vi "sv_Harmonic Distortion and Noise.vi"(0 "complex spectrum":T11={"complex spectrum response"={"f0"=0.0, "df"=1.0, "complex spectrum"=[]}, "spectrum info"={"channel name"="", "description"="", "x-axis units"=0, "spectral info"={"spectrum type"=enum."Power [Magnitude^2]", "linear/dB"=enum."linear", "window"=0, "window size"=0, "FFT size"=0}, "engineering units"=0, "custom label"="", "dB reference [EU]"=0.0, "peak units"=enum."rms", "weighting filter"=0, "spectral density?"=FALSE, "unit label"="", "spectrum skewed?"=FALSE, "complimentary spectrum units"=enum."none"}} {"spectrum info"."x-axis units" items=["Time (s)"=0, "Frequency-CB (Hz)"=1, "Frequency-CPB (Hz)"=1248, "Frequency-Arbitrary (Hz)"=2357, "Quefrency (s)"=2, "Revolutions (rev)"=3, "Order"=4, "Speed (RPM)"=11, "Speed (rad/s)"=21, "Index"=65535]; "spectrum info"."weighting filter" items=["Linear", "A-weighting", "B-weighting", "C-weighting", "ITU-R 468-4", "Dolby", "CCITT", "C-message", "Wb", "Wc", "Wd", "We", "Wf", "Wh", "Wj", "Wk", "Wm", "AES17 20 kHz lowpass", "AES17 40 kHz lowpass", "AES17 20 kHz highpass", "AES17 40 kHz highpass"]; "spectrum info"."dB reference [EU]" format="%.2f"; "spectrum info"."engineering units" items=["custom..."=0, "V"=1, "A"=21, "C"=30, "pC"=31, "s"=32, "-"=29, "Pa"=2, "N"=20, "g"=3, "m/s^2"=4, "m/s"=5, "m"=6, "mm/s"=12, "mm"=13, "micron/s"=14, "micron"=15, "in/s^2"=7, "in/s"=8, "in"=9, "mil/s"=10, "mil"=11, "rad/s^2"=16, "rad/s"=17, "rad"=18, "deg/s^2"=26, "deg/s"=27, "deg"=28, "RPM"=22, "cycle/s^2"=23, "Hz"=24, "cycle"=25, "strain"=19]; "spectrum info"."spectral info"."window" items=["None "=0, "Hanning"=1, "Hamming"=2, "Blackman-Harris"=3, "Exact Blackman"=4, "Blackman"=5, "Flat Top"=6, "4 Term B-Harris "=7, "7 Term B-Harris"=8, "Low Sidelobe"=9, "Force - Exponential"=10, "Gaussian"=62]; "complex spectrum response"."complex spectrum" format="%.2f"; "complex spectrum response"."df" format="%.2f"; "complex spectrum response"."f0" format="%.2f"}, 3 "frequency range":T4={"start frequency"=-1.0, "stop frequency"=-1.0} {"stop frequency" format="%.2f"; "start frequency" format="%.2f"}, 4 "advanced span [Hz]":dbl=-1.0 format="%.2f", 5 "error in":errorcluster, 8 "maximum harmonic":i32=5, 9 "approx. fund. freq. (optional)":dbl=-1.0 format="%.2p") -> (10 "actual maximum harmonic":i32=5, 11 "detected fundamental frequency":dbl=nan format="%.3p", 12 "frequency range string":string, 13 "detected amplitude":dbl=nan format="%.3p", 15 "distortion measurements":T2={"SINAD [ratio]"=nan, "THD+N [ratio]"=nan, "THD"=nan} {"THD" format="%.3p"; "THD+N [ratio]" format="%.3p"; "SINAD [ratio]" format="%.3p"}, 16 "energy":T1={"total"=nan, "fundamental"=nan, "noise and harmonics"=nan, "harmonic energy"=nan, "noise"=nan} {"noise" format="%.3p"; "harmonic energy" format="%.3p"; "noise and harmonics" format="%.3p"; "fundamental" format="%.3p"; "total" format="%.3p"}, 17 "harmonic components":T3(array[cluster]) {"detected amplitude" format="%.2f"; "detected frequency [Hz]" format="%.2f"}, 19 "error out":errorcluster)   [LabVIEW 2017, in "SoundVib_Distortion.lvlib"]
uses:
  <vilib>/addons/Sound and Vibration/svt_Distortion/SoundVib_Distortion.lvlib
  <vilib>/addons/_NISVFA/_Shared subVIs/Controls/svc_Spectrum Info.ctl
  <vilib>/addons/_NISVFA/_Shared subVIs/Controls/svc_X-Axis Units.ctl
  <vilib>/addons/_NISVFA/_Shared subVIs/Controls/svc_Spectrum Type.ctl
  <vilib>/addons/_NISVFA/_Shared subVIs/Controls/svc_Engineering Units Text Ring.ctl
  <vilib>/addons/_NISVFA/_Shared subVIs/Controls/svc_Weighting Filter Text Ring.ctl
  <vilib>/addons/_NISVFA/_Shared subVIs/Controls/svc_Complimentary Spectrum Units.ctl
  <vilib>/Analysis/BLAS.llb/nrm2 - Vector 2-Norm.vi
  <vilib>/Analysis/BLAS.llb/dznrm2 - Vector 2-Norm (CDB).vi
  <vilib>/addons/_NISVFA/_Shared subVIs/Common/svc_Convert Start and Stop to Start Index and Length.vi
  <vilib>/addons/_NISVFA/_Shared subVIs/Common/svc_Window Parameters.vi
  <vilib>/addons/_NISVFA/_Spectrum Processing/subVIs/svfa_Spectrum Info Window to windowTd Type Def.vi
  <vilib>/addons/_NISVFA/_Spectrum Processing/SVFA Get Spectrum Subset (Complex) (1 Ch).vi
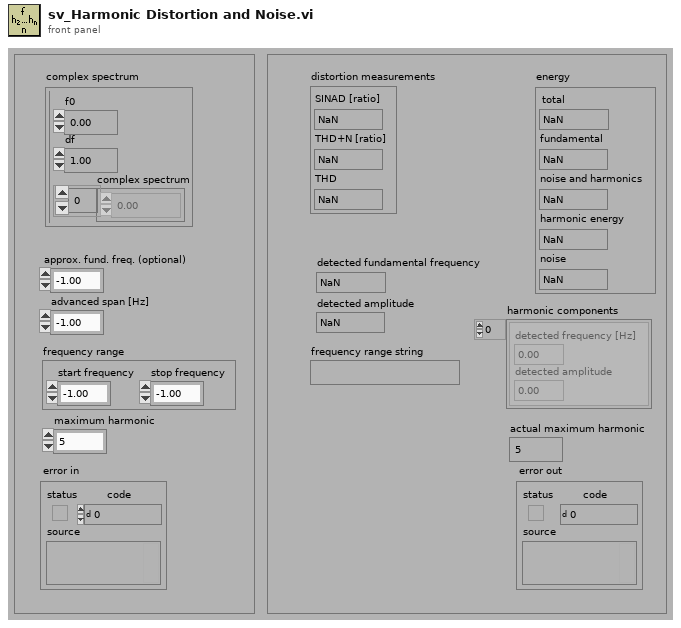
[diagram p1: front panel]
types:
  T1 = cluster{"total":dbl, "fundamental":dbl, "noise and harmonics":dbl, "harmonic energy":dbl, "noise":dbl}
  T2 = cluster{"SINAD [ratio]":dbl, "THD+N [ratio]":dbl, "THD":dbl}
  T3 = cluster{"detected frequency [Hz]":dbl, "detected amplitude":dbl}[]
  T4 = cluster{"start frequency":dbl, "stop frequency":dbl}
  T5 = typedef "svc_Spectrum Info.ctl" = cluster{"channel name":string, "description":string, "x-axis units":T6, "spectral info":cluster{"spectrum type":T7, "linear/dB":enum16{"linear", "dB"}, "window":u16, "window size":i32, "FFT size":i32}, "engineering units":T8, "custom label":string, "dB reference [EU]":dbl, "peak units":enum16{"rms", "peak", "peak-peak"}, "weighting filter":T9, "spectral density?":bool, "unit label":string, "spectrum skewed?":bool, "complimentary spectrum units":T10}
  T6 = typedef "svc_X-Axis Units.ctl" = u16
  T7 = typedef "svc_Spectrum Type.ctl" = enum16{"FFT Spectrum [complex]", "Amplitude [Magnitude]", "Power [Magnitude^2]", "Cross Spectrum [complex]", "Frequency Response [Complex]"}
  T8 = typedef "svc_Engineering Units Text Ring.ctl" = u16
  T9 = typedef "svc_Weighting Filter Text Ring.ctl" = u16
  T10 = typedef "svc_Complimentary Spectrum Units.ctl" = enum16{"none", "radians", "degrees", "cycles", "imaginary"}
  T11 = cluster{"complex spectrum response":cluster{"f0":dbl, "df":dbl, "complex spectrum":cdb[]}, "spectrum info":T5}
  T12 = enum32{"none", "input signal", "detected signal", "residual signal"}
  T13 = cluster{"complex spectrum subset":cluster{"x0":dbl, "dx":dbl, "complex array":cdb[]}, "spectrum info":T5}
  T14 = cluster{"detected frequency [Hz]":dbl, "detected amplitude":dbl}
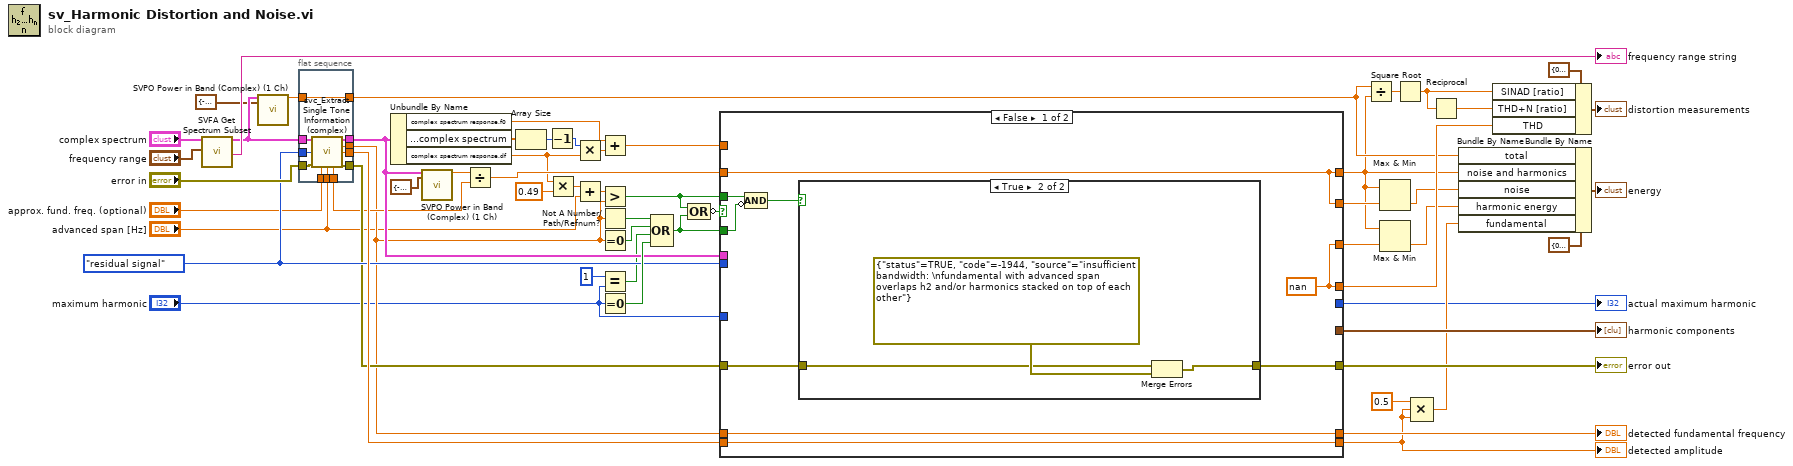
[diagram p0: block diagram]
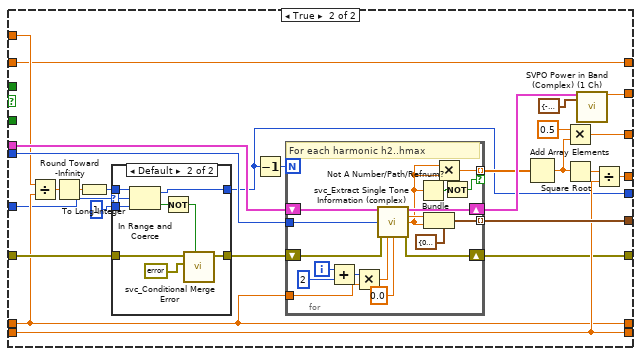
[diagram p3: hidden frame]
diagram:
  w34 = T12."residual signal" ("export signals")
  n1 = call-poly <vilib>:"SVFA Get Spectrum Subset.vi"("complex spectrum"="complex spectrum", "range"="frequency range") -> ("complex spectrum subset"=w28:T13, "range label"=→"frequency range string":string)  [unwired: 14 in, 2 out]
  n2 = call <vilib>:"SVPO Power in Band (Complex) (1 Ch).vi"("complex spectrum"=w28, "range"=cluster{"start":dbl, "stop":dbl} {"start"=-1.0, "stop"=-1.0}) -> ("power in band [EU^2 rms]"=w31:dbl)  [unwired: 17 in]
  n3 = flat-sequence {
    tunnel: "error in" -> [w69]
    tunnel: "approx. fund. freq. (optional)" -> [w68]
    tunnel: [w67] -> w26
    tunnel: w28 -> [w66]
    tunnel: w34 -> [w65]
    tunnel: [w64] -> w27
    tunnel: [w63] -> w14
    tunnel: [w62] -> w43
    tunnel: "advanced span [Hz]" -> [w61]
    tunnel: w31 -> [w60]
    tunnel: [w60] -> w30
    tunnel: [w59] -> w25
    frame #0 {
      n4 = call <vilib>:"svc_Extract Single Tone Information (complex).vi"("complex spectrum"=w66, "export signals"=w65, "error in"=w69, "approximate frequency [Hz]"=w68, "advanced span [Hz]"=w61) -> ("complex spectrum"=w64:T11, "frequency [Hz]"=w63:dbl, "amplitude [EU pk]"=w62:dbl, "residual bandwidth ratio"=w59:dbl, "error out"=w67:errorcluster)  [unwired: 5 in, 1 out]
    }
  }
  n5 = Unbundle By Name(w27) -> ("complex spectrum response.f0"=w20:dbl, "complex spectrum response.complex spectrum"=w40:cdb[], "complex spectrum response.df"=w5:dbl)
  n6 = call <vilib>:"SVPO Power in Band (Complex) (1 Ch).vi"("complex spectrum"=w27, "range"=cluster{"start":dbl, "stop":dbl} {"start"=-1.0, "stop"=-1.0}) -> ("power in band [EU^2 rms]"=w24:dbl)  [unwired: 17 in]
  n7 = Divide(x=w24, y=w25) -> (x/y=w21:dbl)
  n8 = Array Size(array=w40) -> (size(s)=w3:i32)
  n9 = Decrement(x=w3) -> (x-1=w2:i32)
  n10 = Multiply(x=w5, y=0.49) -> (x*y=w4:dbl)
  n11 = Multiply(x=w2, y=w5) -> (x*y=w23:dbl)
  n12 = Add(x=w4, y="advanced span [Hz]") -> (x+y=w53:dbl)
  n13 = Add(x=w20, y=w23) -> (x+y=w22:dbl)
  n14 = Greater?(x=w53, y=w14) -> (0:w7:bool)
  n15 = Not A Number/Path/Refnum?(number/path/refnum=w14) -> (NaN/Path/Refnum?=w56:bool)
  n16 = Equal To 0?(x=w14) -> (x = 0?=w52:bool)
  n17 = Equal?(x=1, y="maximum harmonic") -> (x = y?=w10:bool)
  n18 = Equal To 0?(x="maximum harmonic") -> (x = 0?=w51:bool)
  n19 = Compound Arithmetic op=OR(w56, w52, w10, w51) -> (w15:bool)
  n20 = Compound Arithmetic op=OR(w7, w15) -> (invert w16:bool)
  n21 = case shown="False" w16 {
    tunnel: [w71 w108] -> w46
    tunnel: w43 -> [w75 w90]
    tunnel: w26 -> [w78 w107]
    tunnel: [_ w106] -> w55
    tunnel: "maximum harmonic" -> [_ w83]
    tunnel: [w77 w86] -> w54
    tunnel: w27 -> [_ w105]
    tunnel: w14 -> [w76 w88]
    tunnel: w7 -> [w73 _]
    tunnel: [w71 w104] -> w38
    tunnel: [w70 w103] -> w36
    tunnel: w34 -> [_ w102]
    tunnel: w21 -> [w70 w91]
    tunnel: [_ w84] -> w35
    tunnel: w22 -> [_ w92]
    tunnel: [w76 w88] -> w19
    tunnel: [w75 w90] -> w18
    tunnel: [w70 w91] -> w17
    tunnel: w15 -> [w74 _]
    frame False {
      w71 = nan
      n22 = Compound Arithmetic op=AND(w73, invert w74) -> (w72:bool)
      n23 = case shown="True" w72 {
        tunnel: w78 -> [w79 w81]
        tunnel: [w79 w80] -> w77
        frame False {
          # "The detected frequency is NaN iff the input complex spectrum is empty.\nThe detected frequency is zero if the input complex spectrum is zeros.\nWe do not change the error status as we prefer not to throw errors if a \nVI is run with default parameters."
        }
        frame True {
          n24 = Merge Errors(w81, errorcluster {"status"=TRUE, "code"=-1944, "source"="insufficient bandwidth: \nfundamental with advanced span overlaps h2 and/or harmonics stacked on top of each other"} ("error out")) -> (w80:errorcluster)
        }
      }
    }
    frame True {
      n25 = Divide(x=w92, y=w88) -> (x/y=w101:dbl)
      n26 = Round Toward -Infinity(1:w101) -> (0:w99:dbl)
      n27 = To Long Integer(number=w99) -> (32bit integer=w100:i32)
      n28 = case shown="Default" w83 {
        selector: w83 -> [_ w118]
        tunnel: w100 -> [w110 w119]
        tunnel: [w110 w117] -> w84
        tunnel: w107 -> [w109 w113]
        tunnel: [w109 w112] -> w94
        tunnel: 1 ("lower limit") -> [_ w116]
        frame -1 {
        }
        frame Default {
          n29 = In Range and Coerce(upper limit=w119, x=w118, lower limit=w116) -> (coerced(x)=w117:i32, In Range?=w115:bool)
          n30 = Not(x=w115) -> (.not. x?=w114:bool)
          n31 = call <vilib>:"svc_Conditional Merge Error.vi"("merge"=w114, "new error"=errorcluster {"status"=FALSE, "code"=1946, "source"="max harmonic coerced"} ("error out"), "error in (no error)"=w113) -> ("error out"=w112:errorcluster)  [unwired: 8 in]
        }
      }
      n32 = Decrement(x=w84) -> (x-1=w98:i32)
      n33 = for {
        N: w98 -> [_]
        tunnel: [w124] -> w85 mode=indexing if=w120
        tunnel: [w137] -> w106 mode=indexing
        tunnel: w102 -> [w134]
        shift-right: [w135] -> w93
        shift-left: w105 -> [w136]
        tunnel: w88 -> [w130]
        shift-right: [w125] -> w86
        shift-left: w94 -> [w126]
        i -> [w131]
        # "For each harmonic h2..hmax"
        n34 = Add(x=w131, y=2) -> (x+y=w129:i32)
        n35 = Multiply(x=w129, y=w130) -> (x*y=w127:dbl)
        n36 = call <vilib>:"svc_Extract Single Tone Information (complex).vi"("complex spectrum"=w136, "export signals"=w134, "error in"=w126, "approximate frequency [Hz]"=w127, "advanced span [Hz]"=0.0) -> ("complex spectrum"=w135:T11, "frequency [Hz]"=w123:dbl, "amplitude [EU pk]"=w122:dbl, "error out"=w125:errorcluster)  [unwired: 5 in, 2 out]
        n37 = Not A Number/Path/Refnum?(number/path/refnum=w122) -> (NaN/Path/Refnum?=w121:bool)
        n38 = Bundle(cluster=T14 {"detected frequency [Hz]"=0.0, "detected amplitude"=0.0}, "detected frequency [Hz]"=w123, "detected amplitude"=w122) -> (w137:T14)
        n39 = Multiply(x=w122, y=w122) -> (x*y=w124:dbl)
        n40 = Not(x=w121) -> (.not. x?=w120:bool)
      }
      n41 = Add Array Elements(numeric array=w85) -> (sum=w96:dbl)
      n42 = Multiply(x=0.5, y=w96) -> (x*y=w104:dbl)
      n43 = Square Root(x=w96) -> (sqrt(x)=w97:dbl)
      n44 = call <vilib>:"SVPO Power in Band (Complex) (1 Ch).vi"("complex spectrum"=w93, "range"=cluster{"start":dbl, "stop":dbl} {"start"=-1.0, "stop"=-1.0}) -> ("power in band [EU^2 rms]"=w103:dbl)  [unwired: 17 in]
      n45 = Divide(x=w97, y=w90) -> (x/y=w108:dbl)
    }
  }
  "error out" <- w54
  "detected fundamental frequency" <- w19
  "detected amplitude" <- w18
  "harmonic components" <- w55
  "actual maximum harmonic" <- w35
  n46 = Divide(x=w30, y=w17) -> (x/y=w58:dbl)
  n47 = Max & Min(x=w17, y=w36) -> (min(x,y)=w37:dbl)  [unwired: 1 out]
  n48 = Max & Min(x=w17, y=w38) -> (min(x,y)=w39:dbl)  [unwired: 1 out]
  n49 = Square Root(x=w58) -> (sqrt(x)=w48:dbl)
  n50 = Compound Arithmetic op=MULTIPLY(0.5 ("value"), w18, w18) -> (w42:dbl)
  n51 = Reciprocal(x=w48) -> (1/x=w47:dbl)
  n52 = Bundle By Name(cluster=T1 {"total"=0.0, "fundamental"=0.0, "noise and harmonics"=0.0, "harmonic energy"=0.0, "noise"=0.0} ("energy"), "total"=w30, "noise and harmonics"=w17, "noise"=w37, "harmonic energy"=w39, "fundamental"=w42) -> (→"energy":T1)
  n53 = Bundle By Name(cluster=T2 {"SINAD [ratio]"=0.0, "THD+N [ratio]"=0.0, "THD"=0.0} ("distortion measurements"), "SINAD [ratio]"=w48, "THD+N [ratio]"=w47, "THD"=w46) -> (→"distortion measurements":T2)
